vi "Set print Offset.vi"(8 "error in (no error)":errorcluster, 11 "Domino Laser module Class in":refnum<class "Domino Laser module Class.lvclass">) -> (0 "error out":errorcluster, 3 "Domino Laser module Class out":refnum<class "Domino Laser module Class.lvclass">)   [LabVIEW 2015, in "Domino LM.lvlib" / "Domino Laser module Class.lvclass"]
uses:
  CTRLS/Domino Laser module Class.lvclass
  CTRLS/Domino Laser module Class.lvclass/Domino Laser module Class.ctl
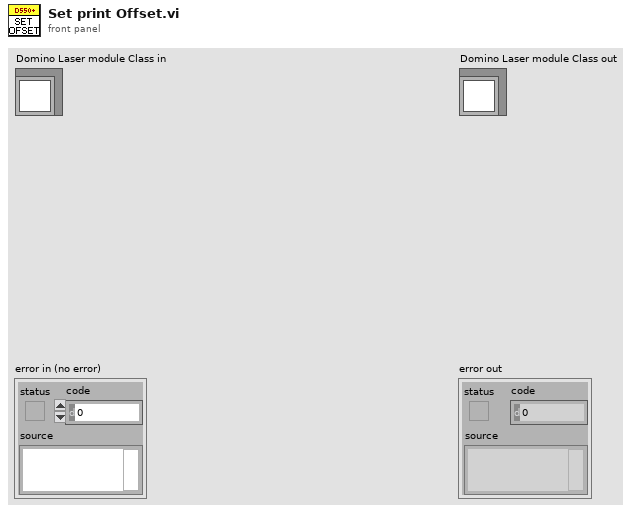
[diagram p1: front panel]
types:
  T1 = cluster{"Camera Offset [MM]":u32, "Reject Offset [MM]":u32, "Reject Delay [% of Width]":u32, "Carton Width [MM]":u32, "Carton Width Error [MM] ":u16, "Reject Verify Offset [MM]":u32, "Gate Width B [MM] \n":u32, "Printer offset X":i16, "Printer offset Y":i16}
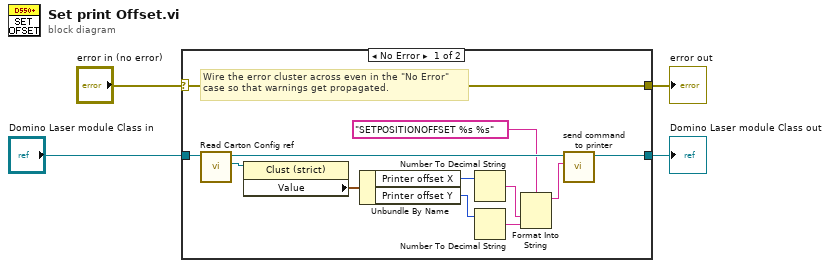
[diagram p0: block diagram]
diagram:
  n1 = case shown="No Error" "error in (no error)" {
    selector: "error in (no error)" -> [w16 w18]
    tunnel: [w16 w18] -> w3
    tunnel: [w15 w17] -> w1
    tunnel: "Domino Laser module Class in" -> [w14 w17]
    frame No Error {
      # "Wire the error cluster across even in the \"No Error\"\ncase so that warnings get propagated."
      n2 = call "Read Carton Config ref.vi"("Domino Laser module Class in"=w14) -> ("Carton Config"=w12:refnum<vi>, "Domino Laser module Class out"=w13:refnum<class "Domino Laser module Class.lvclass">)  [unwired: 8 in, 1 out]
      n3 = property class="Clust (strict)"(reference=w12) -> ("Value"=w11:T1)  [unwired: 1 in, 2 out]
      n4 = Unbundle By Name(w11) -> ("Printer offset X"=w10:i16, "Printer offset Y"=w9:i16)
      n5 = Number To Decimal String(number=w10) -> (decimal integer string=w8:string)  [unwired: 1 in]
      n6 = Number To Decimal String(number=w9) -> (decimal integer string=w7:string)  [unwired: 1 in]
      n7 = Format Into String(format string="SETPOSITIONOFFSET %s %s", w8, w7) -> (resulting string=w5:string)  [unwired: 2 in, 1 out]
      n8 = call "send command to printer.vi"("command to be sent"=w5, "Domino Laser module Class in"=w13) -> ("Domino Laser module Class out"=w15:refnum<class "Domino Laser module Class.lvclass">)  [unwired: 6 in, 3 out]
    }
    frame Error {
    }
  }
  "error out" <- w3
  "Domino Laser module Class out" <- w1
